vi "Close Channels.vi"(8 "error in (no error)":errorcluster, 9 "Channel List(\"\")":string, 11 "VISA resource name":refnum<visa-resource-name>) -> (0 "error out":errorcluster, 3 "VISA resource name out":refnum<visa-resource-name>)   [LabVIEW 2024, in "Keithley DMM6500 DAQ6500 Series.lvlib"]
doc: "Closes the listed channels without affecting any other channels."
uses:
  Keithley DMM6500 DAQ6500 Series.lvlib
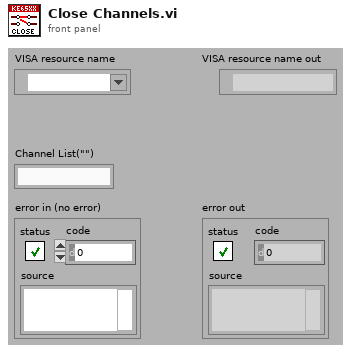
[diagram p1: front panel]
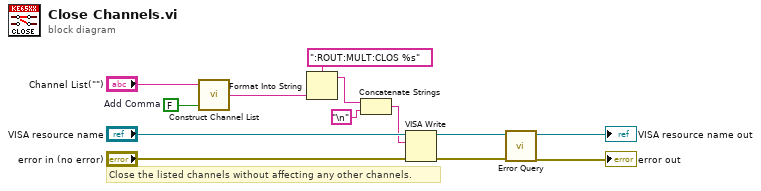
[diagram p0: block diagram]
diagram:
  w4 = FALSE  # Add Comma
  # "Close the listed channels without affecting any other channels."
  n1 = call "Construct Channel List.vi"("Add Comma (True)"=w4, "Channel List"="Channel List(\"\")") -> ("Channel List String"=w6:string)  [unwired: 1 in]
  n2 = Format Into String(format string=":ROUT:MULT:CLOS %s", w6) -> (resulting string=w2:string)  [unwired: 2 in, 1 out]
  n3 = Concatenate Strings(w2, "\n") -> (w3:string)
  n4 = VISA Write(VISA resource name="VISA resource name", write buffer=w3, error in (no error)="error in (no error)") -> (VISA resource name out=w10:refnum<visa-resource-name>, error out=w9:errorcluster)  [unwired: 1 out]
  n5 = call "Error Query.vi"("error in (no error)"=w9, "VISA resource name"=w10) -> ("error out"=→"error out":errorcluster, "VISA resource name out"=→"VISA resource name out":refnum<visa-resource-name>)  [unwired: 6 in, 2 out]
